vi "Read.vi"(8 "error in (no error)":errorcluster, 11 "TimeStamper in":refnum<class "TimeStamper.lvclass">) -> (0 "error out":errorcluster, 1 "Messages":T1(array[cluster]), 2 "Timestamps":T2(array[cluster]), 3 "TimeStamper out":refnum<class "TimeStamper.lvclass">)   [LabVIEW 2011, in "TimeStamper.lvclass"]
uses:
  TimeStamper.lvclass
  TimeStamper.lvclass/TimeStamper.ctl
  CounterTimestamp.ctl
  <vilib>/DAQmx/read.llb/DAQmx Read (Counter U32 1Chan 1Samp).vi
  <vilib>/DAQmx/miscellaneous.llb/DAQmx Fill In Error Info.vi
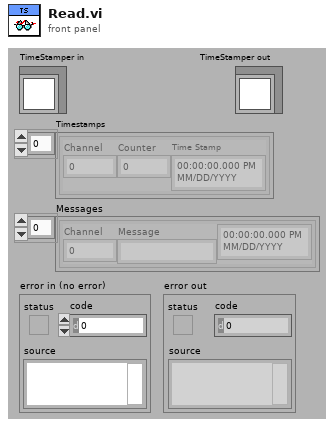
[diagram p1: front panel]
types:
  T1 = cluster{"Channel":dbl, "Message":string, timestamp}[]
  T2 = cluster{"Channel":i32, "Counter":u32, "Time Stamp":timestamp}[]
  T3 = typedef "TimeStamper.lvclass/CounterTimestamp.ctl" = cluster{"Channel":u8, "Counter":u32, "Time Stamp":timestamp}
  T4 = cluster{"Channel":i32, "Counter Value":u32, "seconds since 1Jan1904":timestamp}
  T5 = cluster{"Channel":i32, "Counter Value":u32, "seconds since 1Jan1904":timestamp}[]
  T6 = cluster{"Channel":u8, "Message":string, "Time Stamp":timestamp}
  T7 = cluster{"Channel":dbl, "Message":string, "Time Stamp":timestamp}[]
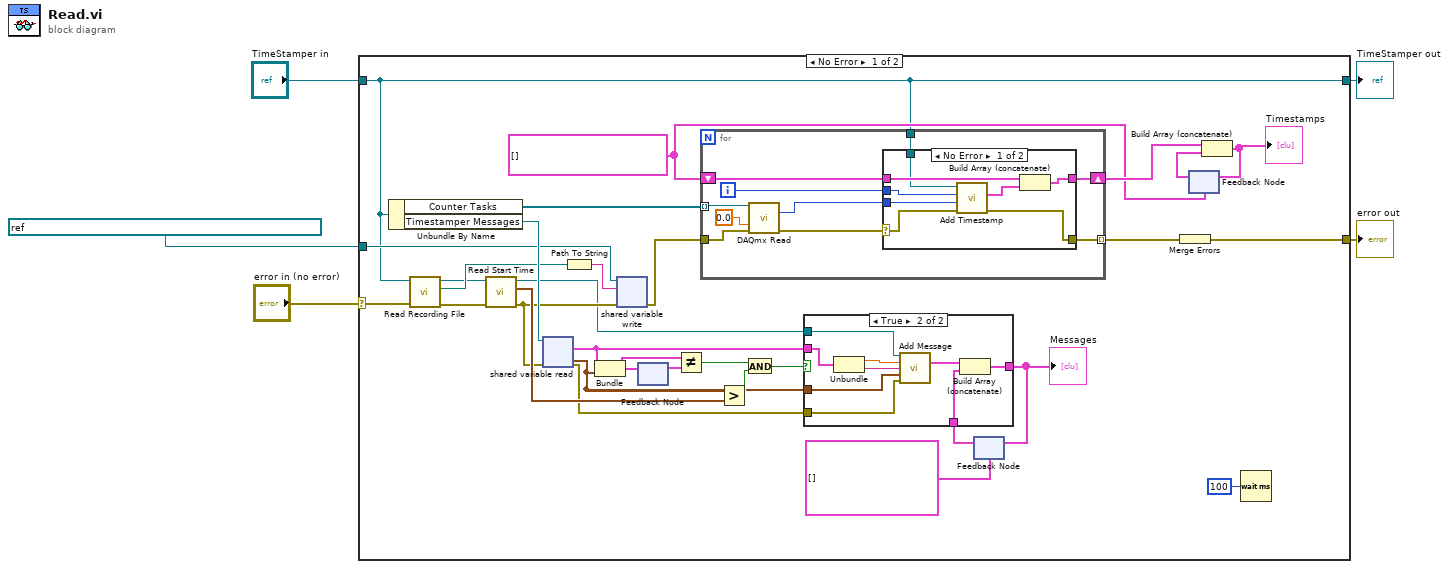
[diagram p0: block diagram]
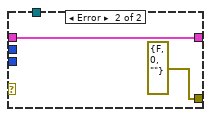
[diagram p3: hidden frame]
diagram:
  n1 = case shown="No Error" "error in (no error)" {
    selector: "error in (no error)" -> [w19 w68]
    tunnel: [w6 w68] -> w4
    tunnel: [w16 w67] -> w2
    tunnel: "TimeStamper in" -> [w16 w67]
    tunnel: refnum<k21> "ni.var.psp://My Computer/AcquisitionVariables/SessionPath" ("shared variable refnum in") -> [w28 _]
    frame No Error {
      w27 = T3[] []
      n2 = Unbundle By Name(w16) -> ("Counter Tasks"=w36:refnum<k21>[], "Timestamper Messages"=w31:refnum<k21>)
      n3 = call-dynamic "Read Recording File.vi"("error in (no error)"=w19, "AcquistionObject in"=w16) -> ("error out"=w15:errorcluster, "Recording File"=w20:path, "AcquistionObject out"=w17:refnum<class "TimeStamper.lvclass">)  [unwired: 7 in]
      n4 = call-dynamic "Read Start Time.vi"("error in (no error)"=w15, "AcquistionObject in"=w17) -> ("error out"=w14:errorcluster, "Start Time"=w21:timestamp, "AcquistionObject out"=w13:refnum<class "TimeStamper.lvclass">)  [unwired: 7 in]
      n5 = shared-variable-read(w31, w14) -> (w12:errorcluster, w9:cluster{dbl, string}, w11:timestamp)  [unwired: 1 out]
      n6 = Path To String(path=w20) -> (string=w29:string)
      n7 = Bundle(w9, w11) -> (w10:cluster{cluster{dbl, string}, timestamp})  [unwired: 1 in]
      n8 = shared-variable-write(w28, w14, w29) -> (w18:errorcluster)  [unwired: 1 out]
      n9 = feedback-in #1(w10) -> ()
      n10 = feedback #1() -> (w30:cluster{cluster{dbl, string}, timestamp})  [unwired: 1 in]
      n11 = Not Equal?(x=w10, y=w30) -> (x != y?=w8:bool)
      n12 = for {
        tunnel: w36 -> [w56] mode=indexing
        shift-right: [w51] -> w34
        shift-left: w27 -> [w50]
        tunnel: w16 -> [w47]
        tunnel: w18 -> [w55]
        tunnel: [w48] -> w7 mode=indexing
        i -> [w53]
        n13 = call-poly <vilib>:"DAQmx Read.vi"("task/channels in"=w56, "timeout"=0.0, "error in"=w55) -> ("data"=w52:u32, "error out"=w49:errorcluster)  [unwired: 10 in, 1 out]
        n14 = case shown="No Error" w49 {
          selector: w49 -> [w61 _]
          tunnel: w53 -> [w63 _]
          tunnel: w52 -> [w62 _]
          tunnel: w50 -> [w64 w66]
          tunnel: [w57 w66] -> w51
          tunnel: [w58 errorcluster {"status"=FALSE, "code"=0, "source"=""} ("error IO")] -> w48
          tunnel: w47 -> [w59 _]
          frame No Error {
            n15 = call-dynamic "Add Timestamp.vi"("error in (no error)"=w61, "Counter Value"=w62, "Channel"=w63, "TimeStamper in"=w59) -> ("error out"=w58:errorcluster, "Timestamp"=w60:T4)  [unwired: 5 in, 1 out]
            n16 = Build Array (concatenate)(w64, w60) -> (w57:T5)
          }
          frame Error {
          }
        }
      }
      n17 = Greater?(x=w11, y=w21) -> (0:w24:bool)
      n18 = And(x=w8, y=w24) -> (x .and. y?=w23:bool)
      n19 = feedback #2(T1 []) -> (w26:T1)
      n20 = case shown="True" w23 {
        tunnel: w9 -> [_ w46]
        tunnel: w11 -> [_ w40]
        tunnel: [w37 w45] -> w25
        tunnel: w26 -> [w37 w44]
        tunnel: w13 -> [_ w39]
        tunnel: w12 -> [_ w38]
        frame False {
        }
        frame True {
          n21 = Unbundle(w46) -> (w42:dbl, w41:string)
          n22 = call-dynamic "Add Message.vi"("TimeStamper in"=w39, "Channel"=w42, "Message"=w41, "Time Stamp"=w40, "error in (no error)"=w38) -> ("Cluster"=w43:T6)  [unwired: 8 in, 2 out]
          n23 = Build Array (concatenate)(w43, w44) -> (w45:T7)
        }
      }
      "Messages" <- w25
      n24 = feedback-in #2(w25) -> ()
      n25 = Merge Errors(w7) -> (w6:errorcluster)
      n26 = feedback #3(w27) -> (w33:T2)
      n27 = Build Array (concatenate)(w34, w33) -> (w32:T2)
      "Timestamps" <- w32
      n28 = feedback-in #3(w32) -> ()
      n29 = Wait (ms)(milliseconds to wait=u32 100) -> ()  [unwired: 1 out]
    }
    frame Error {
    }
  }
  "error out" <- w4
  "TimeStamper out" <- w2
